vi "Get Commd.vi"(8 "error in (no error)":errorcluster, 11 "Channel in":refnum<class "Channel.lvclass">) -> (0 "error out":errorcluster, 3 "Channel out":refnum<class "Channel.lvclass">)   [LabVIEW 2018, in "Channel.lvclass"]
doc: "Remove from the qeue the last command sent by the control interface"
uses:
  Channel.lvclass
  Channel.lvclass/Channel.ctl
  Log File/CCS_Log File.lvclass
  RxTx/CCS_RxTx.lvclass
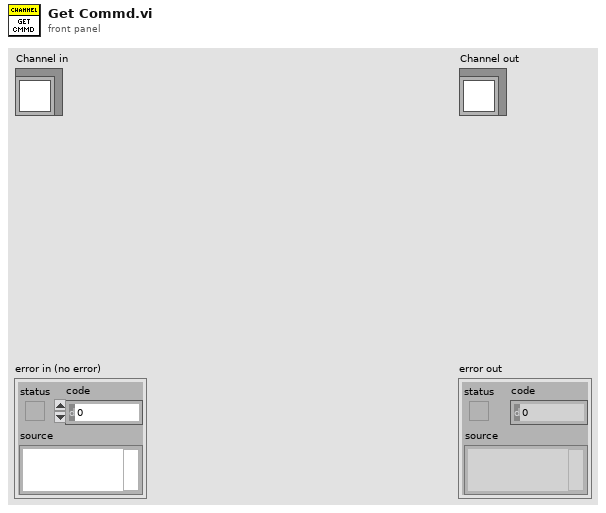
[diagram p1: front panel]
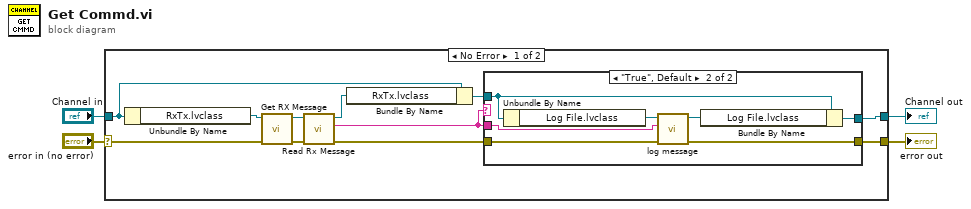
[diagram p0: block diagram]
diagram:
  n1 = case shown="No Error" "error in (no error)" {
    selector: "error in (no error)" -> [w14 w26]
    tunnel: [w10 w26] -> w3
    tunnel: [w11 w25] -> w1
    tunnel: "Channel in" -> [w13 w25]
    frame No Error {
      n2 = Unbundle By Name(w13) -> ("RxTx.lvclass"=w15:refnum<class "CCS_RxTx.lvclass">)
      n3 = call "Get RX Message.vi"("error in (no error)"=w14, "RxTx in"=w15) -> ("error out"=w9:errorcluster, "RxTx out"=w6:refnum<class "CCS_RxTx.lvclass">)  [unwired: 7 in, 1 out]
      n4 = call "Read Rx Message.vi"("error in (no error)"=w9, "RxTx in"=w6) -> ("error out"=w8:errorcluster, "Rx Message"=w5:string, "RxTx out"=w7:refnum<class "CCS_RxTx.lvclass">)  [unwired: 7 in]
      n5 = Bundle By Name(cluster=w13, "RxTx.lvclass"=w7) -> (w12:refnum<class "Channel.lvclass">)
      n6 = case shown="\"True\", Default" w5 {
        tunnel: w12 -> [w17 w24]
        tunnel: [w17 w23] -> w11
        tunnel: [w16 w20] -> w10
        tunnel: w8 -> [w16 w19]
        tunnel: w5 -> [_ w18]
        frame "" {
        }
        frame "True", Default {
          n7 = Unbundle By Name(w24) -> ("Log File.lvclass"=w22:refnum<class "CCS_Log File.lvclass">)
          n8 = call-dynamic "log message.vi"("error in (no error)"=w19, "Message to log"=w18, "Log File in"=w22) -> ("error out"=w20:errorcluster, "Log File out"=w21:refnum<class "CCS_Log File.lvclass">)  [unwired: 7 in]
          n9 = Bundle By Name(cluster=w24, "Log File.lvclass"=w21) -> (w23:refnum<class "Channel.lvclass">)
        }
      }
    }
    frame Error {
    }
  }
  "error out" <- w3
  "Channel out" <- w1
